vi "Add Logging Section.vi"(8 "error in":errorcluster, 11 "Ballard MIL-STD 1553 custom device in":T1 format="%.0x") -> (0 "error out":errorcluster, 2 "logging":T1 format="%.0x", 3 "Ballard MIL-STD 1553 custom device out":T1 format="%.0x")   [LabVIEW 2020, in "Ballard MIL-STD-1553 Scripting.lvlib"]
uses:
  Ballard MIL-STD-1553 Scripting.lvlib
  <vilib>/NI VeriStand/Custom Device API/Custom Device Item Ref.ctl
  Constants.vi
  <vilib>/NI VeriStand/Custom Device API/Custom Device API.lvlib
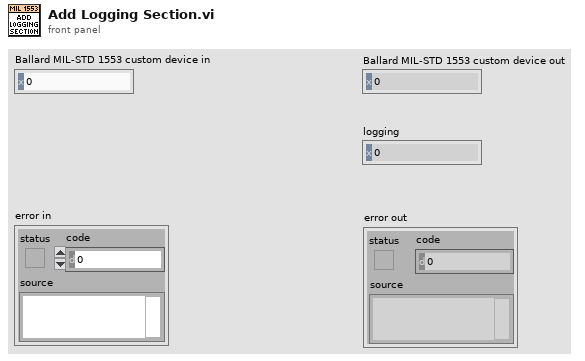
[diagram p1: front panel]
types:
  T1 = typedef "Custom Device API.lvlib/Custom Device Item Ref.ctl" = u64
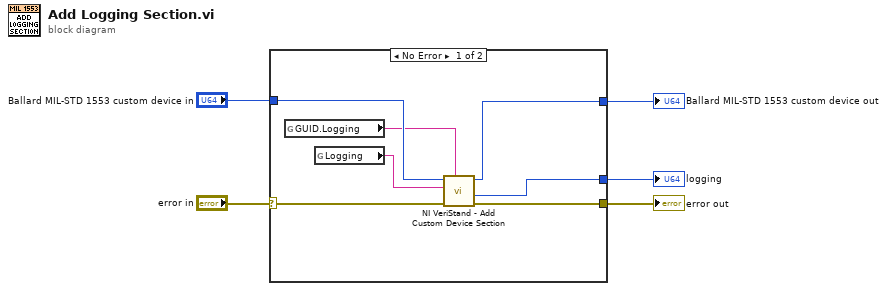
[diagram p0: block diagram]
diagram:
  n1 = case shown="No Error" "error in" {
    selector: "error in" -> [w11 w14]
    tunnel: "Ballard MIL-STD 1553 custom device in" -> [w12 w13]
    tunnel: [w9 w14] -> w4
    tunnel: [w10 w13] -> w3
    tunnel: [w8 _] -> w1
    frame No Error {
      n2 = global read "Constants.vi" "GUID.Logging"() -> (w7:string)
      n3 = global read "Constants.vi" "Logging"() -> (w6:string)
      n4 = call <vilib>:"NI VeriStand - Add Custom Device Section.vi"("GUID (Default Section)"=w7, "error in (no error)"=w11, "Section Name"=w6, "Parent Ref in"=w12) -> ("error out"=w9:errorcluster, "Section Ptr"=w8:T1, "Parent Ref out"=w10:T1)  [unwired: 4 in, 1 out]
    }
    frame Error {
    }
  }
  "error out" <- w4
  "Ballard MIL-STD 1553 custom device out" <- w3
  "logging" <- w1
